vi "AGGIORNA LISTA PROFILI.vi"(8 "error in (no error)":errorcluster, 9 "FILTRA PER TIPO":bool, 10 "TIPO":string, 11 "Refnum in":T1) -> (0 "error out":errorcluster, 2 "Array":string[](array[string]), 3 "Refnum out":T1)   [LabVIEW 2019]
uses:
  <vilib>/addons/database/Connection.llb/Conn ObjectReference.ctl
  <vilib>/addons/database/NI_Database_API.lvlib
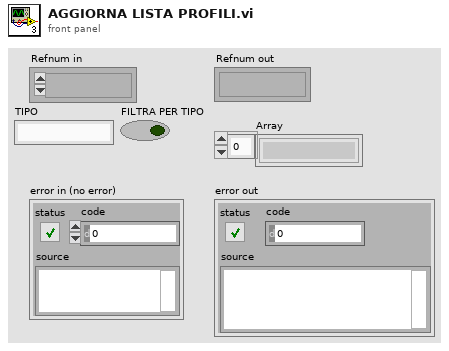
[diagram p1: front panel]
types:
  T1 = typedef "NI_Database_API.lvlib/Conn ObjectReference.ctl" = refnum<k1>
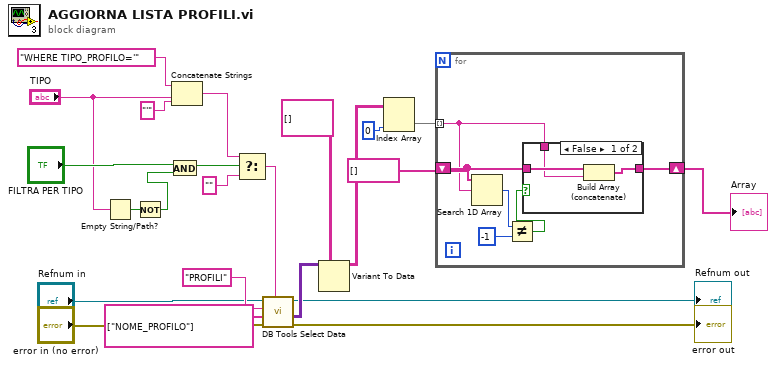
[diagram p0: block diagram]
diagram:
  n1 = Empty String/Path?(string/path="TIPO") -> (empty?=w5:bool)
  n2 = Not(x=w5) -> (.not. x?=w3:bool)
  n3 = And(x="FILTRA PER TIPO", y=w3) -> (x .and. y?=w4:bool)
  n4 = Concatenate Strings("WHERE TIPO_PROFILO='" ("condition"), "TIPO", "'" ("string")) -> (w10:string)
  n5 = Select(t=w10, s=w4, f="") -> (s? t:f=w9:string)
  n6 = call <vilib>:"DB Tools Select Data.vi"("condition"=w9, "error in (no error)"="error in (no error)", "columns"=string[] ["NOME_PROFILO"], "table"="PROFILI", "connection reference"="Refnum in") -> ("error out"=→"error out":errorcluster, "data"=w16:variant[][], "connection reference out"=→"Refnum out":T1)  [unwired: 1 in]
  n7 = Variant To Data(type=string[][] [] ("Item Names"), Variant=w16) -> (data=w21:string[][])  [unwired: 1 in, 1 out]
  n8 = Index Array(array=w21, index (col)=0 ("disabled index (col)")) -> (element=w23:string[])  [unwired: 1 in]
  n9 = for {
    tunnel: w23 -> [w27] mode=indexing
    shift-right: [w29] -> w1
    shift-left: string[] [] -> [w28]
    n10 = Search 1D Array(1D array=w28, element=w27) -> (index of element=w26:i32)  [unwired: 1 in]
    n11 = Not Equal?(x=w26, y=-1) -> (x != y?=w24:bool)
    n12 = case shown="False" w24 {
      tunnel: w28 -> [w32 w33]
      tunnel: [w31 w33] -> w29
      tunnel: w27 -> [w30 _]
      frame False {
        n13 = Build Array (concatenate)(w32, w30) -> (w31:string[])
      }
      frame True {
      }
    }
  }
  "Array" <- w1
